vi "SwitchWavelength.vi"() -> ()   [LabVIEW 2009]
panel:
  in  "Use Polarizers":bool
  in  "Mode":enum16{"K band", "H band"}(ring)
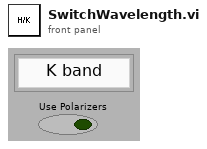
[diagram p1: front panel]
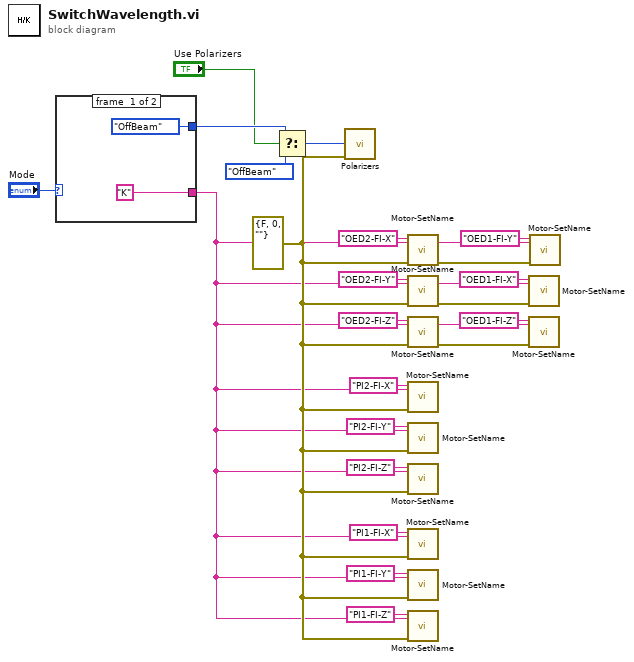
[diagram p0: block diagram]
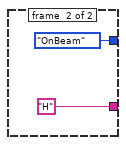
[diagram p2: hidden frame]
diagram:
  w6 = errorcluster {"status"=FALSE, "code"=0, "source"=""} ("error in (no error)")
  n1 = case shown="\"H band\"" "Mode" {
    tunnel: ["K" "H"] -> w5
    tunnel: [enum16{"OnBeam", "OffBeam"}."OffBeam" ("Polarizers State") enum16{"OnBeam", "OffBeam"}."OnBeam" ("Polarizers State")] -> w3
    frame #0 {
    }
    frame #1 {
    }
  }
  n2 = Select(t=w3, s="Use Polarizers", f=enum16{"OnBeam", "OffBeam"}."OffBeam") -> (s? t:f=w4:enum16{"OnBeam", "OffBeam"})
  n3 = call "Polarizers.vi"("Polarizers State"=w4, "error in (no error)"=w6) -> ()  [unwired: 8 out]
  n4 = call "Motor-SetName.vi"("Name"=w5, "Motor"="OED2-FI-X", "error in (no error)"=w6) -> ("error out"=w12:errorcluster)  [unwired: 6 out]
  n5 = call "Motor-SetName.vi"("Name"=w5, "Motor"="OED2-FI-Y", "error in (no error)"=w6) -> ("error out"=w8:errorcluster)  [unwired: 6 out]
  n6 = call "Motor-SetName.vi"("Name"=w5, "Motor"="OED2-FI-Z", "error in (no error)"=w6) -> ("error out"=w7:errorcluster)  [unwired: 6 out]
  n7 = call "Motor-SetName.vi"("Name"=w5, "Motor"="PI2-FI-X", "error in (no error)"=w6) -> ()  [unwired: 7 out]
  n8 = call "Motor-SetName.vi"("Name"=w5, "Motor"="PI2-FI-Y", "error in (no error)"=w6) -> ()  [unwired: 7 out]
  n9 = call "Motor-SetName.vi"("Name"=w5, "Motor"="PI2-FI-Z", "error in (no error)"=w6) -> ()  [unwired: 7 out]
  n10 = call "Motor-SetName.vi"("Name"=w5, "Motor"="PI1-FI-X", "error in (no error)"=w6) -> ()  [unwired: 7 out]
  n11 = call "Motor-SetName.vi"("Name"=w5, "Motor"="PI1-FI-Y", "error in (no error)"=w6) -> ()  [unwired: 7 out]
  n12 = call "Motor-SetName.vi"("Name"=w5, "Motor"="PI1-FI-Z", "error in (no error)"=w6) -> ()  [unwired: 7 out]
  n13 = call "Motor-SetName.vi"("Name"=w5, "Motor"="OED1-FI-X", "error in (no error)"=w8) -> ()  [unwired: 7 out]
  n14 = call "Motor-SetName.vi"("Name"=w5, "Motor"="OED1-FI-Z", "error in (no error)"=w7) -> ()  [unwired: 7 out]
  n15 = call "Motor-SetName.vi"("Name"=w5, "Motor"="OED1-FI-Y", "error in (no error)"=w12) -> ()  [unwired: 7 out]
